vi "入栈.vi"(8 "error in (no error)":errorcluster caption="错误输入（无错误）", 10 "元素":dbl, 11 "堆栈(DBL) 输入":refnum<class "堆栈(DBL).lvclass"> caption="DNL_LabVIEW Object in") -> (0 "error out":errorcluster caption="错误输出", 3 "堆栈(DBL) 输出":refnum<class "堆栈(DBL).lvclass"> caption="DNL_LabVIEW Object out")   [LabVIEW 2011, in "堆栈(DBL).lvclass"]
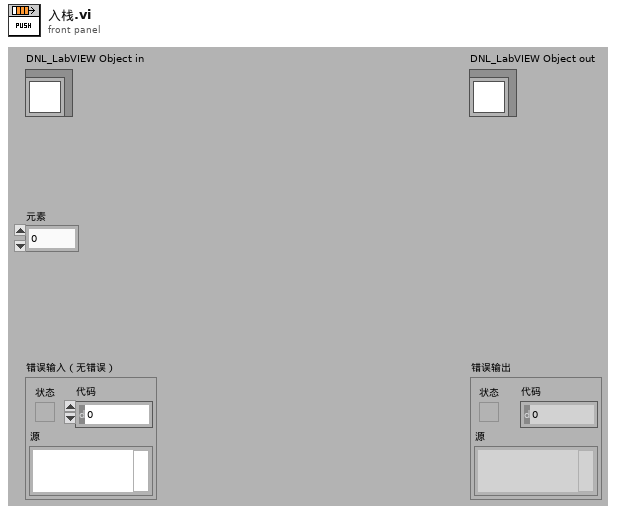
[diagram p1: front panel]
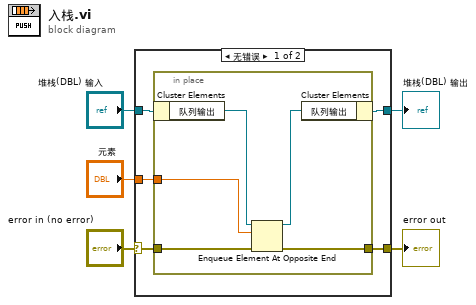
[diagram p0: block diagram]
diagram:
  n1 = case shown="无错误" "error in (no error)" {
    selector: "error in (no error)" -> [w7 w17]
    tunnel: [w6 w17] -> w4
    tunnel: [w9 w16] -> w2
    tunnel: "堆栈(DBL) 输入" -> [w10 w16]
    tunnel: "元素" -> [w8 _]
    frame No Error {
      n2 = in-place {
        in-place-border: w8 -> [w13]
        in-place-border: w7 -> [w12]
        in-place-border: [w11] -> w6
        n3 = in-place-cluster #1(w10) -> ("队列输出"=w15:refnum<queue>)
        n4 = Enqueue Element At Opposite End(queue=w15, element=w13, error in (no error)=w12) -> (queue out=w14:refnum<queue>, error out=w11:errorcluster)  [unwired: 1 in, 1 out]
        n5 = in-place-cluster #1("队列输出"=w14) -> (w9:refnum<class "堆栈(DBL).lvclass">)
      }
    }
    frame Error {
    }
  }
  "error out" <- w4
  "堆栈(DBL) 输出" <- w2
